vi "Monitor Viewer.vi"() -> ()   [LabVIEW 2015]
panel:
  out "text 2":string[](array[string])
  out "text":string
  in  "Log file":path=path "C:/Data/Shot Log.txt"
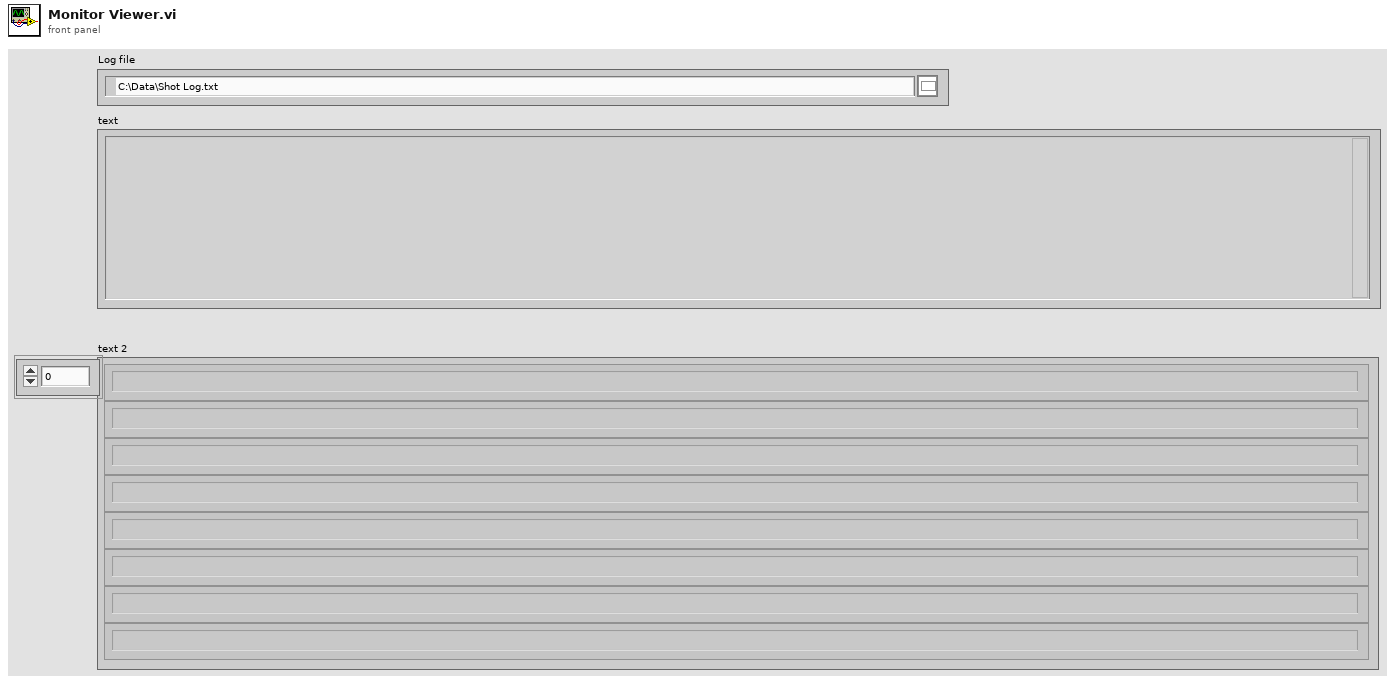
[diagram p1: front panel]
types:
  T1 = enum16{"open", "replace", "create", "open or create", "replace or create", "replace or create with confirmation"}
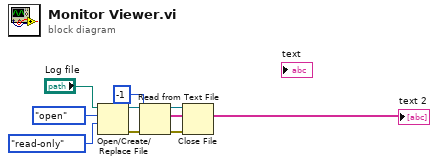
[diagram p0: block diagram]
diagram:
  n1 = Open/Create/Replace File(file path (use dialog)="Log file", operation (0:open)=T1."open", access (0:read/write)=enum16{"read/write", "read-only", "write-only"}."read-only") -> (refnum out=w8:refnum<file>, error out=w3:errorcluster)  [unwired: 3 in, 1 out]
  n2 = Read from Text File(file (use dialog)=w8, count=-1, error in=w3) -> (refnum out=w4:refnum<file>, text=→"text 2":string[], error out=w5:errorcluster)  [unwired: 1 in, 1 out]
  n3 = Close File(refnum=w4, error in=w5) -> ()  [unwired: 2 out]
